vi "TEMOCR-Initialize Analysis.vi"(0 "Expt State":T3, 5 "Params":T5, 11 "error in (no error)":errorcluster, 13 "controls":T4) -> (4 "State":T1, 8 "Analysis":T2, 15 "error out":errorcluster)   [LabVIEW 2015]
uses:
  Typedefs/TEMOCR-Parameters.ctl
  Typedefs/TEMOCR-Probe.ctl
  Typedefs/TEMOCR-Elicitor.ctl
  Human Studies/SFM Frontend/LV Source/Typedefs/HSTS-Transducer.ctl
  Typedefs/TEMOCR-Sequence.ctl
  Typedefs/TEMOCR-Analysis.ctl
  Typedefs/TEMOCR-Controls.ctl
  CFTS Main Panel SubVIs/CFTS-Experiment State.ctl
  Typedefs/TEMOCR-Analysis State.ctl
  Utility VIs/Math VIs/dB to Linear (scalar).vi
  Utility VIs/Math VIs/LinSpace (start-stop-step).vi
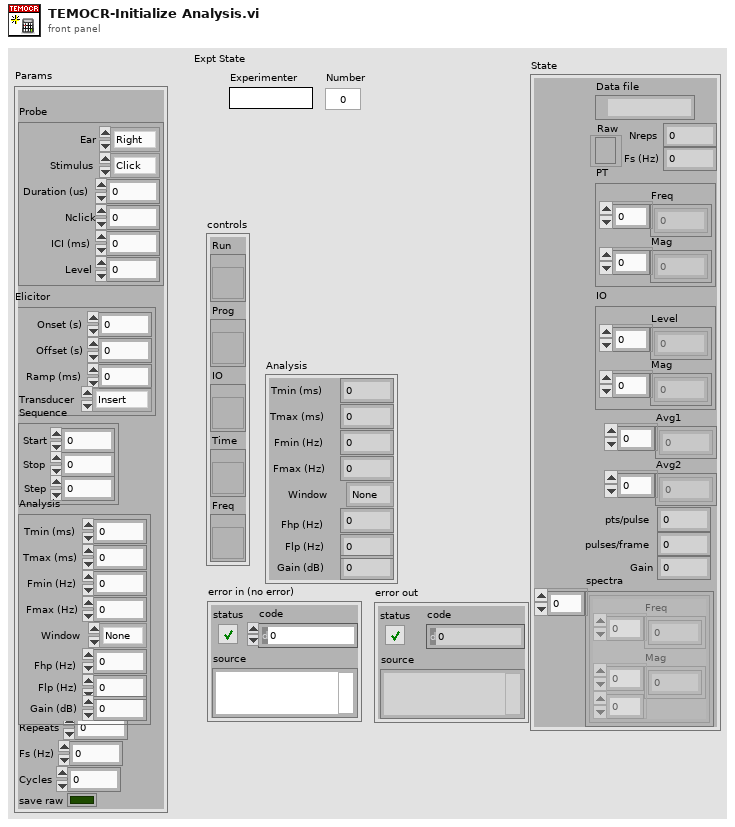
[diagram p1: front panel]
types:
  T1 = typedef "TEMOCR-Analysis State.ctl" = cluster{"Data file":path, "Raw":refnum<file>, "PT":cluster{"Freq":dbl[], "Mag":dbl[]}, "IO":cluster{"Level":dbl[], "Mag":dbl[]}, "Nreps":i32, "Fs (Hz)":dbl, "Avg1":dbl[], "pts/pulse":i32, "pulses/frame":i32, "Avg2":dbl[], "Gain":dbl, "spectra":cluster{"Freq":dbl[], "Mag":dbl[][]}[]}
  T2 = typedef "TEMOCR-Analysis.ctl" = cluster{"Tmin (ms)":dbl, "Tmax (ms)":dbl, "Fmin (Hz)":dbl, "Fmax (Hz)":dbl, "Window":enum16{"None", "Hanning", "Hamming"}, "Fhp (Hz)":dbl, "Flp (Hz)":dbl, "Gain (dB)":dbl}
  T3 = typedef "CFTS-Experiment State.ctl" = cluster{"Experimenter":string, "Number":u32, "Right":string, "Left":string, "Data Folder":path, "State File":path, "Version Info":string, "End Exposure Time":dbl, "Exposure Duration":string, "Run #":cluster{"CAP":i16, "ABR":i16, "DP":i16, "VsEP":i16, "MeasSeq":i16, "SubSeq":i16, "SFOAE":i16}}
  T4 = typedef "TEMOCR-Controls.ctl" = cluster{"Run":refnum<vi>, "Prog":refnum<vi>, "IO":refnum<vi>, "Time":refnum<vi>, "Freq":refnum<vi>}
  T5 = typedef "TEMOCR-Parameters.ctl" = cluster{"Probe":T6, "Elicitor":T7, "Sequence":T9, "Analysis":T2, "Repeats":i32, "Fs (Hz)":dbl, "Cycles":i32, "save raw":bool}
  T6 = typedef "TEMOCR-Probe.ctl" = cluster{"Ear":enum16{"Right", "Left"}, "Stimulus":enum16{"Click", "Chirp"}, "Duration (us)":dbl, "Nclick":i32, "ICI (ms)":dbl, "Level":dbl}
  T7 = typedef "TEMOCR-Elicitor.ctl" = cluster{"Onset (s)":dbl, "Offset (s)":dbl, "Ramp (ms)":dbl, "Transducer":T8}
  T8 = typedef "HSTS-Transducer.ctl" = enum16{"Insert", "TDH-39", "HD300", "ER-10X"}
  T9 = typedef "TEMOCR-Sequence.ctl" = cluster{"Start":dbl, "Stop":dbl, "Step":dbl}
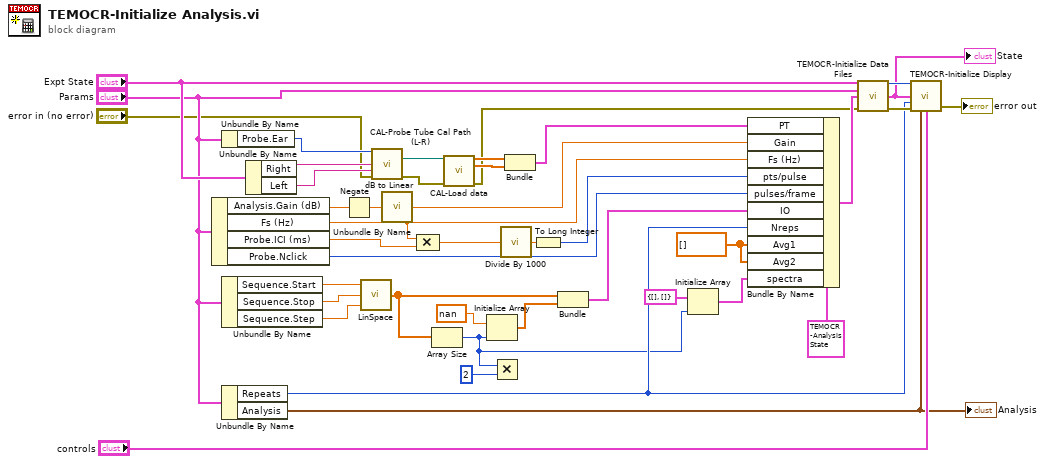
[diagram p0: block diagram]
diagram:
  w11 = dbl[] [] ("Avg")
  n1 = Unbundle By Name("Params") -> ("Analysis.Gain (dB)"=w6:dbl, "Fs (Hz)"=w14:dbl, "Probe.ICI (ms)"=w10:dbl, "Probe.Nclick"=w9:i32)
  n2 = Unbundle By Name("Params") -> ("Probe.Ear"=w39:enum16{"Right", "Left"})
  n3 = Unbundle By Name("Params") -> ("Sequence.Start"=w33:dbl, "Sequence.Stop"=w31:dbl, "Sequence.Step"=w32:dbl)
  n4 = Unbundle By Name("Params") -> ("Repeats"=w7:i32, "Analysis"=w19:T2)
  "Analysis" <- w19
  n5 = Unbundle By Name("Expt State") -> ("Right"=w41:string, "Left"=w40:string)
  n6 = Negate(x=w6) -> (-x=w5:dbl)
  n7 = call-poly "LinSpace.vi"("Step"=w32, "Stop"=w31, "Start"=w33) -> ("Array"=w29:dbl[])  [unwired: 1 in, 1 out]
  n8 = call "CAL-Probe Tube Cal Path (L-R).vi"("Ear"=w39, "Right"=w41, "Left"=w40, "error in (no error)"="error in (no error)") -> ("Probe Tube Cal Path"=w38:path, "error out"=w37:errorcluster)  [unwired: 10 in]
  n9 = call-poly "dB to Linear.vi"("dB"=w5) -> ("linear"=w4:dbl)
  n10 = Compound Arithmetic op=MULTIPLY(w14, w10) -> (w17:dbl)
  n11 = Array Size(array=w29) -> (size(s)=w2:i32)
  n12 = call "CAL-Load data.vi"("user path"=w38, "error in (no error)"=w37) -> ("Frequency (Hz)"=w36:dbl[], "Mag"=w35:dbl[], "error out"=w13:errorcluster)  [unwired: 6 in, 5 out]
  n13 = Initialize Array(nan, w2) -> (w28:dbl[])
  n14 = Multiply(x=w2, y=2) -> ()  [unwired: 1 out]
  n15 = call "Divide By 1000.vi"("X"=w17) -> ("X/1000"=w15:dbl)
  n16 = Bundle("Frequency (Hz)"=w36, "Mag"=w35) -> (w34:cluster{"Frequency (Hz)":dbl[], "Mag":dbl[]})  [unwired: 1 in]
  n17 = To Long Integer(number=w15) -> (32bit integer=w16:i32)
  n18 = Bundle("Array"=w29, w28) -> (w27:cluster{"Array":dbl[], dbl[]})  [unwired: 1 in]
  n19 = Initialize Array(cluster{"Freq":dbl[], "Mag":dbl[][]} {"Freq"=[], "Mag"=[]} ("spectra"), w2) -> (w1:cluster{"Freq":dbl[], "Mag":dbl[][]}[])
  n20 = Bundle By Name(cluster=T1 {"Data file"=path "", "Raw"=refnum, "PT"={"Freq"=[], "Mag"=[]}, "IO"={"Level"=[], "Mag"=[]}, "Nreps"=0, "Fs (Hz)"=0.0, "Avg1"=[], "pts/pulse"=0, "pulses/frame"=0, "Avg2"=[], "Gain"=0.0, "spectra"=[]} ("Analysis State"), "PT"=w34, "Gain"=w4, "Fs (Hz)"=w14, "pts/pulse"=w16, "pulses/frame"=w9, "IO"=w27, "Nreps"=w7, "Avg1"=w11, "Avg2"=w11, "spectra"=w1) -> (w26:T1)
  n21 = call "TEMOCR-Initialize Data Files.vi"("Expt State"="Expt State", "Params"="Params", "State In"=w26, "error in (no error)"=w13) -> ("Run"=w21:i32, "State Out"=w20:T1, "error out"=w24:errorcluster)  [unwired: 9 in]
  "State" <- w20
  n22 = call "TEMOCR-Initialize Display.vi"("Run"=w21, "State"=w20, "Total steps"=w7, "error in (no error)"=w24, "Analysis"=w19, "controls"="controls") -> ("error out"=→"error out":errorcluster)  [unwired: 9 in]
